vi "CRYGet Tree Click State.vi"(10 "Coords":T1, 11 "Tree Ref In":refnum<vi>) -> (0 "In Bounds?":bool, 1 "Row Number":i32, 2 "Tag":string, 3 "Tree Ref Out":refnum<vi>, 4 "In Symbol?":bool, 6 "Symbol":i32)   [LabVIEW 2013]
uses:
  <vilib>/Utility/miscctls.llb/LVPoint32TypeDef.ctl
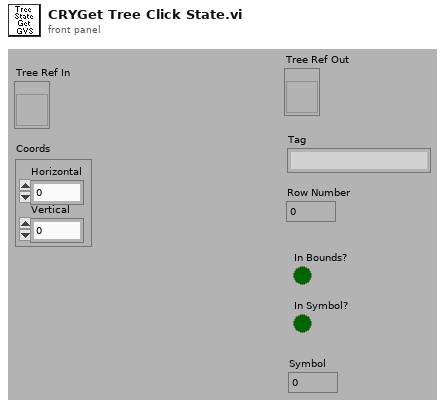
[diagram p1: front panel]
types:
  T1 = typedef "LVPoint32TypeDef.ctl" = cluster{"Horizontal":i32, "Vertical":i32}
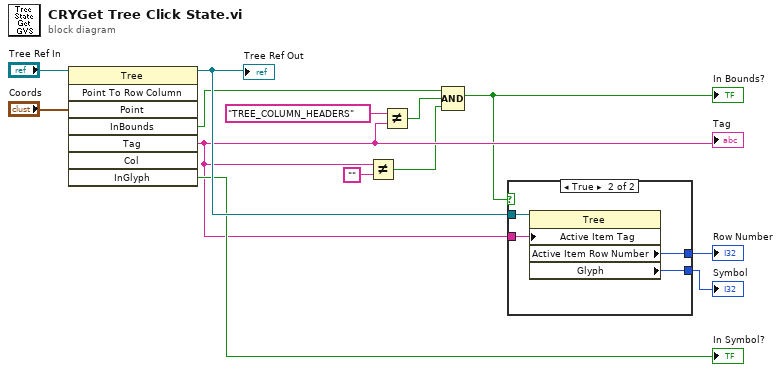
[diagram p0: block diagram]
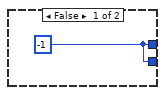
[diagram p2: hidden frame]
diagram:
  n1 = invoke class="Tree" method="Point To Row Column"(reference="Tree Ref In", "Point"="Coords") -> (reference out=w10:refnum<vi>, "InBounds"=w7:bool, "Tag"=w6:string, "InGlyph"=→"In Symbol?":bool)  [unwired: 6 in, 4 out]
  "Tree Ref Out" <- w10
  "Tag" <- w6
  n2 = Not Equal?(x=w6, y="") -> (x != y?=w3:bool)
  n3 = Not Equal?(x="TREE_COLUMN_HEADERS", y=w6) -> (x != y?=w2:bool)
  n4 = Compound Arithmetic op=AND(w7, w2, w3) -> (w1:bool)
  "In Bounds?" <- w1
  n5 = case shown="True" w1 {
    tunnel: [w14 w18] -> w11
    tunnel: w10 -> [_ w17]
    tunnel: w6 -> [_ w16]
    tunnel: [w14 w15] -> w4
    frame False {
      w14 = -1 ("Active Item Row Number")
    }
    frame True {
      n6 = property class="Tree"(reference=w17, "Active Item Tag"=w16) -> ("Active Item Row Number"=w18:i32, "Glyph"=w15:i32)  [unwired: 1 in, 2 out]
    }
  }
  "Row Number" <- w11
  "Symbol" <- w4
